vi "通知2.vi"() -> ()   [LabVIEW 2018]
panel:
  in  "颜色盒":u32(colorbox)
  in  "Reset":bool
  in  "Time":dbl=2.0 format="%#_13g"
  out "字符串":string
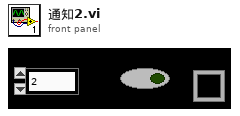
[diagram p1: front panel]
types:
  T1 = typedef "LVRectTypeDef.ctl" = cluster{"Left":i16, "Top":i16, "Right":i16, "Bottom":i16}
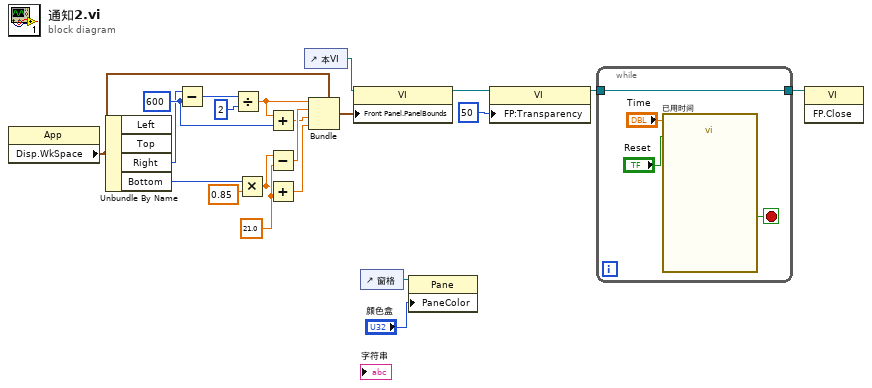
[diagram p0: block diagram]
diagram:
  w14 = 21.0 ("y")
  w7 = i16 600 ("y")
  n1 = property class="App"() -> ("Disp.WkSpace"=w10:T1)  [unwired: 2 in, 2 out]
  n2 = Unbundle By Name(w10) -> ("Right"=w2:i16, "Bottom"=w9:i16)  [unwired: 2 out]
  n3 = Subtract(x=w2, y=w7) -> (x-y=w3:i16)
  n4 = Divide(x=w3, y=i16 2) -> (x/y=w6:dbl)
  n5 = Multiply(x=w9, y=0.85) -> (x*y=w13:dbl)
  n6 = Add(x=w6, y=w7) -> (x+y=w8:dbl)
  n7 = Subtract(x=w13, y=w14) -> (x-y=w15:dbl)
  n8 = Add(x=w13, y=w14) -> (x+y=w16:dbl)
  n9 = control-ref of="本VI"() -> (w5:refnum<vi>)
  n10 = Bundle(cluster=w10, "Left"=w6, "Top"=w15, "Right"=w8, "Bottom"=w16) -> (w11:T1)
  n11 = property class="VI"(reference=w5, "Front Panel.PanelBounds"=w11) -> (reference out=w17:refnum<vi>)  [unwired: 1 in, 1 out]
  n12 = control-ref of="窗格"() -> (w20:refnum<vi>)
  n13 = property class="Pane"(reference=w20, "PaneColor"="颜色盒") -> ()  [unwired: 1 in, 2 out]
  n14 = property class="VI"(reference=w17, "FP:Transparency"=u8 50 ("前面板窗口:透明度")) -> (reference out=w1:refnum<vi>)  [unwired: 1 in, 1 out]
  n15 = while {
    tunnel: [w22] -> w21
    tunnel: w1 -> [w22]
    stop <- w25 stop-if-true
    n16 = call "已用时间"("Time Target (s)"="Time", "Reset"="Reset") -> ("Time has Elapsed"=w25:bool)  [unwired: 10 in, 7 out]
  }
  n17 = invoke class="VI" method="FP.Close"(reference=w21) -> ()  [unwired: 2 in, 3 out]
